vi "Debug.vi"() -> ()   [LabVIEW 2023, in "Panel Actor.lvlib" / "Panel.lvlib" / "Panel Registry.lvclass"]
uses:
  Panel Registry.lvclass
  Static.vi
  Panel Registry.lvclass/Panel Registry.ctl
panel:
  out "Debug Tree":string(tree)
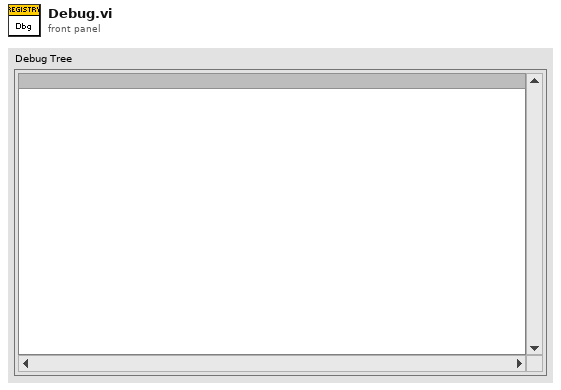
[diagram p1: front panel]
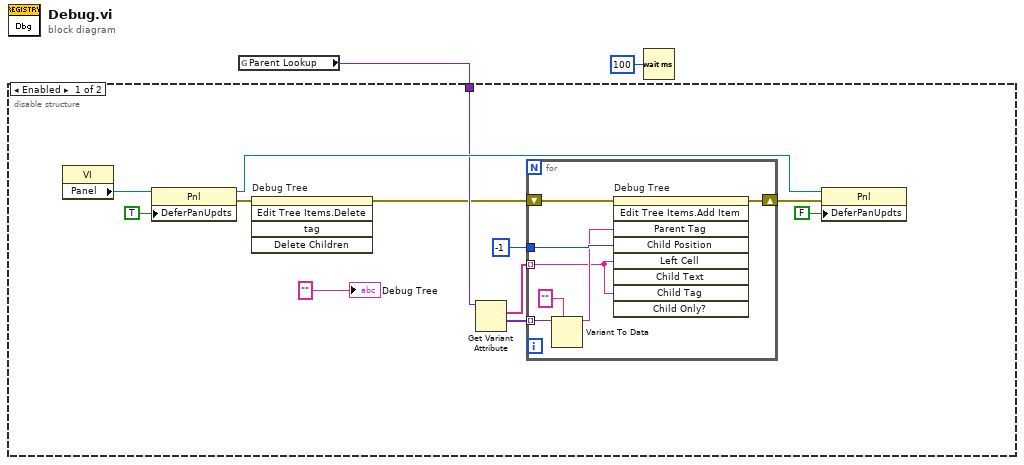
[diagram p0: block diagram]
diagram:
  n1 = global read "Static.vi" "Parent Lookup"() -> (w2:variant)
  n2 = disable-structure shown="Enabled" {
    disable-tunnel: w2 -> [w6 _]
    frame Enabled {
      n3 = property class="VI"() -> ("Panel"=w14:refnum<vi>)  [unwired: 2 in, 2 out]
      n4 = property class="Pnl"(reference=w14, "DeferPanUpdts"=TRUE ("Defer Panel Updates")) -> (reference out=w11:refnum<vi>, error out=w12:errorcluster)  [unwired: 1 in]
      n5 = invoke on="Debug Tree" class="Tree (strict)" method="Edit Tree Items.Delete"(error in=w12) -> (error out=w5:errorcluster)  [unwired: 4 in, 4 out]
      n6 = Get Variant Attribute(Variant=w6) -> (names=w8:string[], values=w7:variant[])  [unwired: 3 in, 2 out]
      n7 = for {
        tunnel: -1 ("Child Position") -> [w21]
        tunnel: w8 -> [w15] mode=indexing
        tunnel: w7 -> [w18] mode=indexing
        shift-right: [w19] -> w4
        shift-left: w5 -> [w20]
        n8 = Variant To Data(type="", Variant=w18) -> (data=w16:string)  [unwired: 1 in, 1 out]
        n9 = invoke on="Debug Tree" class="Tree (strict)" method="Edit Tree Items.Add Item"(error in=w20, "Parent Tag"=w16, "Child Position"=w21, "Left Cell"=w15, "Child Tag"=w15) -> (error out=w19:errorcluster)  [unwired: 4 in, 8 out]
      }
      n10 = property class="Pnl"(reference=w11, error in=w4, "DeferPanUpdts"=FALSE ("Defer Panel Updates")) -> ()  [unwired: 2 out]
      "Debug Tree" <- "" ("Debug Tree")
    }
    frame Disabled {
    }
  }
  n11 = Wait (ms)(milliseconds to wait=u32 100) -> ()  [unwired: 1 out]
